vi "get module information.vi"(8 "error in":errorcluster, 11 "engine mappings":refnum<data-value>) -> (0 "error out":errorcluster, 3 "module info":T1[](array[typedef]))   [LabVIEW 2013, in "PL Framework Configuration Tool.lvlib" / "Engine Mappings.lvclass"]
uses:
  Engine Mappings.lvclass
  module information.ctl
  <vilib>/NI/Tag Bus Module Framework/channel/TBM channel.lvclass
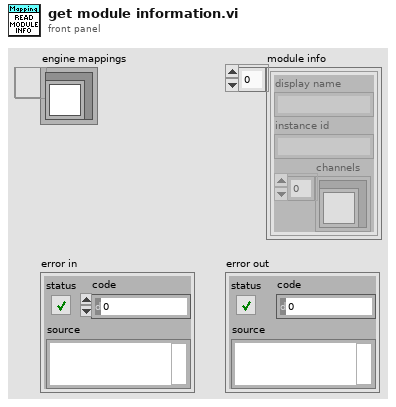
[diagram p1: front panel]
types:
  T1 = typedef "PL Framework Configuration Tool.lvlib/Engine Mappings.lvclass/module information.ctl" = cluster{"display name":string, "instance id":string, "channels":refnum<class "TBM channel.lvclass">[]}
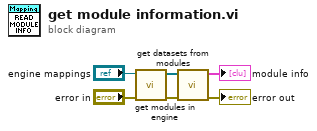
[diagram p0: block diagram]
diagram:
  n1 = call "get modules in engine.vi"("error in"="error in", "engine mapping"="engine mappings") -> ("error out"=w3:errorcluster, "Modules Configurations"=w4:refnum<class "TBM module configuration.lvclass">[])  [unwired: 8 in]
  n2 = call "get datasets from modules.vi"("error in"=w3, "Modules Configurations"=w4) -> ("error out"=→"error out":errorcluster, "module datasets"=→"module info":T1[])  [unwired: 8 in]
